vi "Calibration Audit.vi"() -> ()   [LabVIEW 2014]
doc: "Obtains calibration information for hardware on selected target."
uses:
  <vilib>/Utility/error.llb/DialogType.ctl
  <vilib>/Utility/miscctls.llb/LVRowAndColumnTypeDef.ctl
  <vilib>/nisyscfg/Close (Hardware).vi
  <vilib>/nisyscfg/Close (System).vi
  <vilib>/nisyscfg/Close (Filter).vi
  <vilib>/nisyscfg/nisyscfg.lvlib
  <resource>/objmgr/nisysapi.rc
panel:
  in  "User Name":string
  in  "Password":string
  in  "Target (localhost)":refnum<k21>="localhost"
  out "Calibration Results":string[][](table)
  # "Overview: Obtains calibration information for the hardware on a selected target.\nRequirements: NI System Configuration, applicable device drivers\nInstructions:\n1. Select Target. Enter User Name and Password if necessary.\n2. Run the VI.\n\nThe recommended next calibration date does not account for shelf life. Visit ni.com/calibration to generate an official copy of your NI calibration certificate."
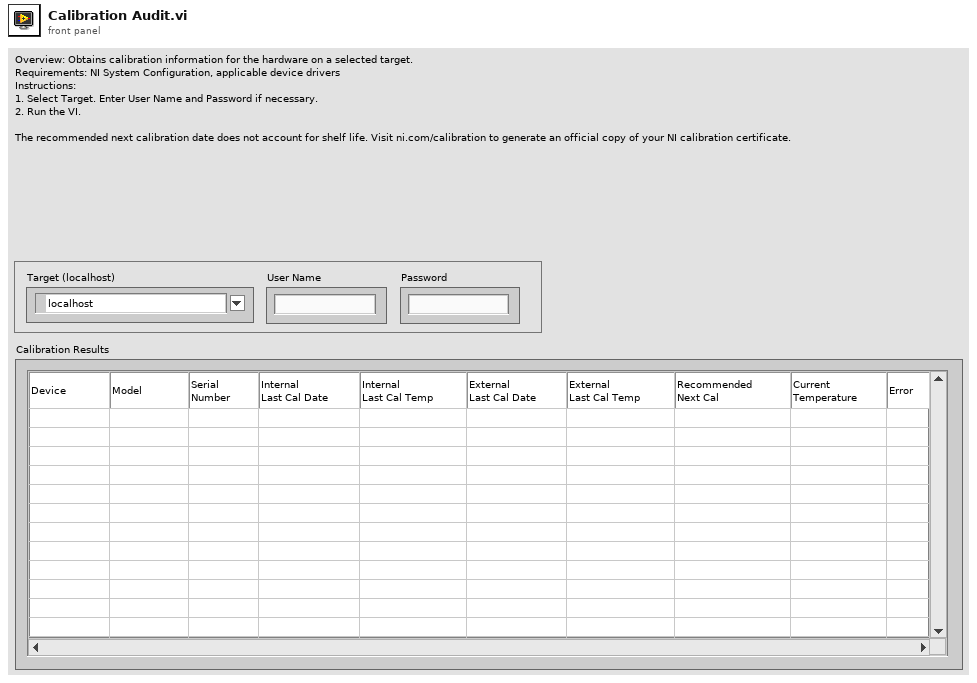
[diagram p1: front panel]
types:
  T1 = typedef "DialogType.ctl" = u16
  T2 = typedef "LVRowAndColumnTypeDef.ctl" = cluster{"Row":i32, "Column":i32}
  T3 = cluster{"Last Calibrated":timestamp, "Last Temperature":dbl, "Recommended Next Calibration":timestamp}
  T4 = cluster{"Last Calibrated":timestamp, "Last Temperature":dbl}
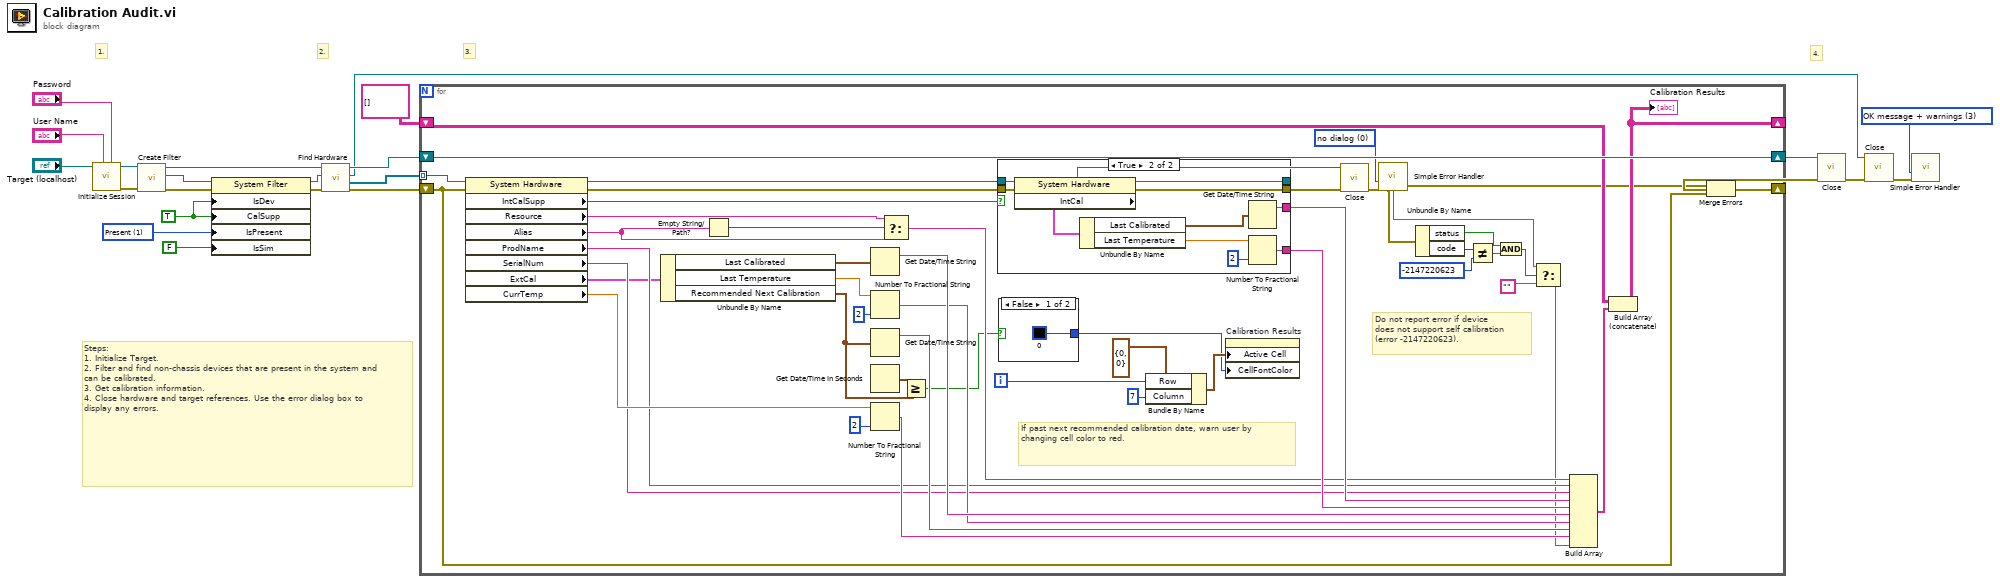
[diagram p0: block diagram]
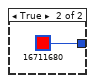
[diagram p3: hidden frame]
diagram:
  w4 = T1 3 items=["no dialog", "OK message", "continue or stop message", "OK message + warnings", "continue/stop + warnings"] ("type of dialog (OK msg:1)")
  w14 = 1 items=["Unknown"=-1, "Not Present"=0, "Present"=1] ("Is Present")
  w21 = TRUE ("Is Device")
  # "3."
  # "4."
  # "2."
  # "1."
  # "Steps:\n1. Initialize Target.\n2. Filter and find non-chassis devices that are present in the system and can be calibrated.\n3. Get calibration information.\n4. Close hardware and target references. Use the error dialog box to display any errors."
  n1 = call <vilib>:"Initialize Session.vi"("Password"="Password", "User Name"="User Name", "Target (localhost)"="Target (localhost)") -> ("error out"=w7:errorcluster, "Session out"=w6:refnum<k21>)  [unwired: 7 in]
  n2 = call <vilib>:"Create Filter.vi"("error in (no error)"=w7, "Session in"=w6) -> ("error out"=w22:errorcluster, "Filter out"=w23:refnum<k20>, "Session out"=w18:refnum<k21>)  [unwired: 7 in]
  n3 = property class="System Filter"(reference=w23, error in=w22, "IsDev"=w21, "CalSupp"=w21, "IsPresent"=w14, "IsSim"=FALSE ("Is Simulated")) -> (reference out=w19:refnum<k20>, error out=w20:errorcluster)
  n4 = call <vilib>:"Find Hardware.vi"("error in (no error)"=w20, "Filter in"=w19, "Session in"=w18) -> ("error out"=w8:errorcluster, "Resources out"=w16:refnum<k20>[], "Filter out"=w9:refnum<k20>, "Session out"=w17:refnum<k21>)  [unwired: 1 in, 4 out]
  n5 = for {
    tunnel: w16 -> [w69] mode=indexing
    shift-right: [w67] -> _
    shift-left: string[][] [] ("appended array") -> [w68]
    shift-right: [w71] -> w10
    shift-left: w17 -> [w71]
    shift-right: [w25] -> w11
    shift-left: w8 -> [w26]
    i -> [w46]
    w45 = T1 0 items=["no dialog", "OK message", "continue or stop message", "OK message + warnings", "continue/stop + warnings"] ("type of dialog (OK msg:1)")
    # "If past next recommended calibration date, warn user by \nchanging cell color to red."
    # "Do not report error if device \ndoes not support self calibration\n(error -2147220623)."
    n6 = property class="System Hardware"(reference=w69, error in=w26) -> (reference out=w33:refnum<k20>, error out=w40:errorcluster, "IntCalSupp"=w34:bool, "Resource"=w35:string, "Alias"=w36:string, "ProdName"=w54:string, "SerialNum"=w53:string, "ExtCal"=w44:T3, "CurrTemp"=w61:dbl)
    n7 = Unbundle By Name(w44) -> ("Last Calibrated"=w38:timestamp, "Last Temperature"=w63:dbl, "Recommended Next Calibration"=w37:timestamp)
    n8 = Empty String/Path?(string/path=w36) -> (empty?=w70:bool)
    n9 = Get Date/Time String(seconds (now)=w38) -> (date string=w58:string)  [unwired: 2 in, 1 out]
    n10 = Number To Fractional String(number=w63, precision (6)=i16 2) -> (F-format string=w57:string)  [unwired: 2 in]
    n11 = Get Date/Time String(seconds (now)=w37) -> (date string=w56:string)  [unwired: 2 in, 1 out]
    n12 = Get Date/Time In Seconds() -> (seconds since 1Jan1904=w47:timestamp)
    n13 = Number To Fractional String(number=w61, precision (6)=i16 2) -> (F-format string=w60:string)  [unwired: 2 in]
    n14 = Select(t=w35, s=w70, f=w36) -> (s? t:f=w55:string)
    n15 = Greater Or Equal?(x=w47, y=w37) -> (x >= y?=w49:bool)
    n16 = case shown="True" w34 {
      tunnel: [_ w83] -> w65
      tunnel: [_ w82] -> w64
      tunnel: [w72 w78] -> w41
      tunnel: w40 -> [w73 w77]
      tunnel: [w73 w76] -> w39
      tunnel: w33 -> [w72 w74]
      frame False {
      }
      frame True {
        n17 = property class="System Hardware"(reference=w74, error in=w77) -> (reference out=w78:refnum<k20>, error out=w76:errorcluster, "IntCal"=w75:T4)
        n18 = Unbundle By Name(w75) -> ("Last Calibrated"=w80:timestamp, "Last Temperature"=w79:dbl)
        n19 = Get Date/Time String(seconds (now)=w80) -> (date string=w83:string)  [unwired: 2 in, 1 out]
        n20 = Number To Fractional String(number=w79, precision (6)=i16 2) -> (F-format string=w82:string)  [unwired: 2 in]
      }
    }
    n21 = case shown="False" w49 {
      tunnel: [u32 0 u32 16711680] -> w50
      frame False {
      }
      frame True {
      }
    }
    n22 = Bundle By Name(cluster=T2 {"Row"=0, "Column"=0} ("Active Cell:Active Cell"), "Row"=w46, "Column"=7) -> (w51:T2)
    n23 = property on="Calibration Results" class="Tbl (strict)"("Active Cell"=w51, "CellFontColor"=w50) -> ()  [unwired: 2 in, 2 out]
    n24 = call-poly <vilib>:"Close.vi"("error in (no error)"=w39, "Resource in"=w41) -> ("error out"=w27:errorcluster)  [unwired: 9 in]
    n25 = call <vilib>:"Simple Error Handler.vi"("type of dialog (OK msg:1)"=w45, "error in (no error)"=w27) -> ("message"=w43:string)  [unwired: 3 in, 4 out]
    n26 = Unbundle By Name(w27) -> ("status"=w31:bool, "code"=w29:i32)
    n27 = Not Equal?(x=w29, y=-2147220623) -> (x != y?=w30:bool)
    n28 = And(x=w31, y=w30) -> (x .and. y?=w32:bool)
    n29 = Select(t=w43, s=w32, f="") -> (s? t:f=w24:string)
    n30 = Build Array(w55, w54, w53, w65, w64, w58, w57, w56, w60, w24) -> (w66:string[])
    n31 = Build Array (concatenate)(w68, w66) -> (w67:string[][])
    "Calibration Results" <- w67
    n32 = Merge Errors(w27, w26) -> (w25:errorcluster)
  }
  n33 = call-poly <vilib>:"Close.vi"("error in (no error)"=w11, "Session in"=w10) -> ("error out"=w12:errorcluster)  [unwired: 9 in]
  n34 = call-poly <vilib>:"Close.vi"("error in (no error)"=w12, "Filter in"=w9) -> ("error out"=w5:errorcluster)  [unwired: 9 in]
  n35 = call <vilib>:"Simple Error Handler.vi"("type of dialog (OK msg:1)"=w4, "error in (no error)"=w5) -> ()  [unwired: 3 in, 5 out]
